vi "Enqueue Change to Cell Cost.vi"(6 "cost":dbl, 8 "error in (no error)":errorcluster, 9 "y":i32, 10 "x":i32, 11 "map reference in":refnum<data-value>) -> (0 "error out":errorcluster, 3 "map reference out":refnum<data-value>)   [LabVIEW 2017, in "NI_Robotics_OccupancyGridWorldMap.lvclass"]
doc: "Requests that LabVIEW update the cost of entering the cell in the occupancy grid map at the <B>x</B>- and <B>y</B>-coordinates you specify."
uses:
  <vilib>/robotics/Navigation/shared/WorldMap/OccupancyGridWorldMap/NI_Robotics_OccupancyGridWorldMap.lvclass
  <vilib>/robotics/Utilities/NI_Robotics Utilities.lvlib
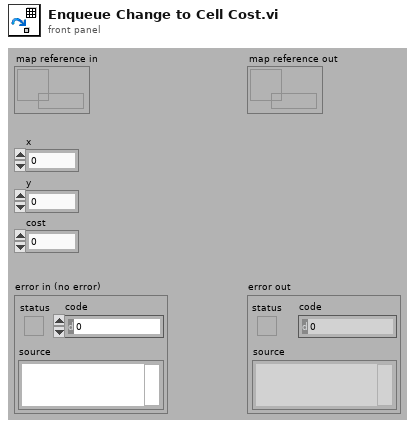
[diagram p1: front panel]
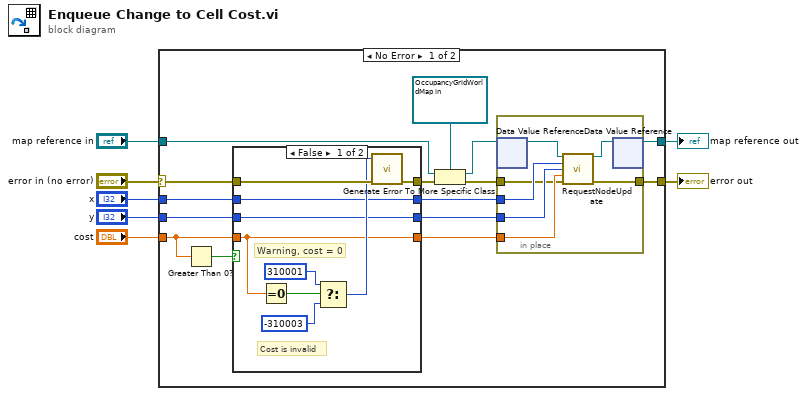
[diagram p0: block diagram]
diagram:
  n1 = case shown="No Error" "error in (no error)" {
    selector: "error in (no error)" -> [w14 w44]
    tunnel: [w22 w43] -> w3
    tunnel: [w21 w44] -> w4
    tunnel: "x" -> [w12 _]
    tunnel: "y" -> [w10 _]
    tunnel: "cost" -> [w8 _]
    tunnel: "map reference in" -> [w18 w43]
    frame No Error {
      n2 = Greater Than 0?(x=w8) -> (x > 0?=w16:bool)
      n3 = case shown="False" w16 {
        tunnel: [w27 w35] -> w15
        tunnel: w14 -> [w28 w35]
        tunnel: [w25 w34] -> w13
        tunnel: w12 -> [w25 w34]
        tunnel: [w24 w33] -> w11
        tunnel: w10 -> [w24 w33]
        tunnel: [w23 w32] -> w9
        tunnel: w8 -> [w23 w32]
        frame False {
          # "Warning, cost = 0"
          # "Cost is invalid"
          n4 = Equal To 0?(x=w23) -> (x = 0?=w31:bool)
          n5 = Select(t=310001 ("code"), s=w31, f=-310003 ("code")) -> (s? t:f=w26:i32)
          n6 = call <vilib>:"Generate Error.vi"("error in (no error)"=w28, "code"=w26) -> ("error out"=w27:errorcluster)  [unwired: 9 in]
        }
        frame True {
        }
      }
      n7 = To More Specific Class(target class=refnum<data-value> refnum ("World Map Reference"), reference=w18, error in=w15) -> (specific class reference=w19:refnum<data-value>, error out=w20:errorcluster)
      n8 = in-place {
        in-place-border: w13 -> [w40]
        in-place-border: w11 -> [w39]
        in-place-border: w9 -> [w38]
        in-place-border: w20 -> [w37]
        in-place-border: [w36] -> w21
        n9 = in-place-dvr #1(w19) -> (w42:refnum<class "NI_Robotics_OccupancyGridWorldMap.lvclass">)  [unwired: 1 out]
        n10 = call-dynamic "RequestNodeUpdate.vi"("OccupancyGridWorldMap in"=w42, "x"=w40, "y"=w39, "Cost"=w38, "error in (no error)"=w37) -> ("OccupancyGridWorldMap out"=w41:refnum<class "NI_Robotics_OccupancyGridWorldMap.lvclass">, "error out"=w36:errorcluster)  [unwired: 9 in]
        n11 = in-place-dvr #1(w41) -> (w22:refnum<data-value>)  [unwired: 1 out]
      }
    }
    frame Error {
    }
  }
  "map reference out" <- w3
  "error out" <- w4
